vi "SubVI Terminals.vi"(6 "Label":string, 8 "error in":errorcluster, 10 "VI":refnum<vi>) -> (0 "error out":errorcluster, 2 "Terminals[]":refnum<vi>[](array[refnum]))   [LabVIEW 2025, in "_Rescript.lvlib"]
uses:
  _Rescript.lvlib
  <vilib>/Utility/traverseref.llb/TRef TravTarget.ctl
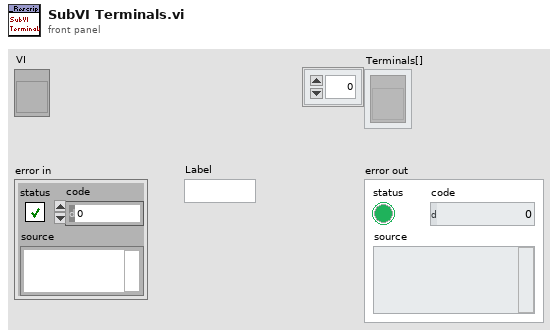
[diagram p1: front panel]
types:
  T1 = typedef "TRef TravTarget.ctl" = enum16{"FP", "BD", "Other"}
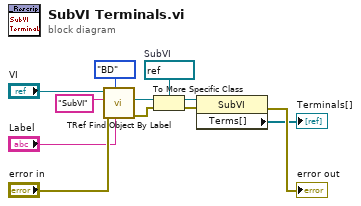
[diagram p0: block diagram]
diagram:
  w11 = refnum<vi> refnum  # SubVI
  n1 = call <vilib>:"TRef Find Object By Label.vi"("Label"="Label", "Traverse Target"=TRef_TravTarget."BD", "error in (no error)"="error in", "Class Name"="SubVI", "VI Ref"="VI") -> ("error out"=w10:errorcluster, "Found Obj Ref"=w6:refnum<vi>)  [unwired: 3 in, 2 out]
  n2 = To More Specific Class(target class=w11, reference=w6, error in=w10) -> (specific class reference=w8:refnum<vi>, error out=w7:errorcluster)
  n3 = property class="SubVI"(reference=w8, error in=w7) -> (error out=→"error out":errorcluster, "Terms[]"=→"Terminals[]":refnum<vi>[])  [unwired: 1 out]
